vi "reserveResources.vi"(8 "error in (no error)":errorcluster, 10 "HWList":string[](array[string]), 11 "HWController in":refnum<class "HWController.lvclass">) -> (0 "error out":errorcluster, 3 "HWController out":refnum<class "HWController.lvclass">)   [LabVIEW 2011, in "Hardware.lvlib" / "HWControllers.lvlib" / "HWController.lvclass"]
uses:
  HWController.lvclass
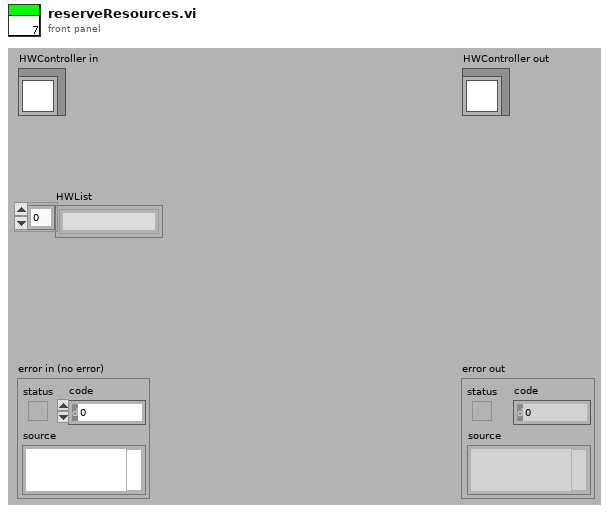
[diagram p1: front panel]
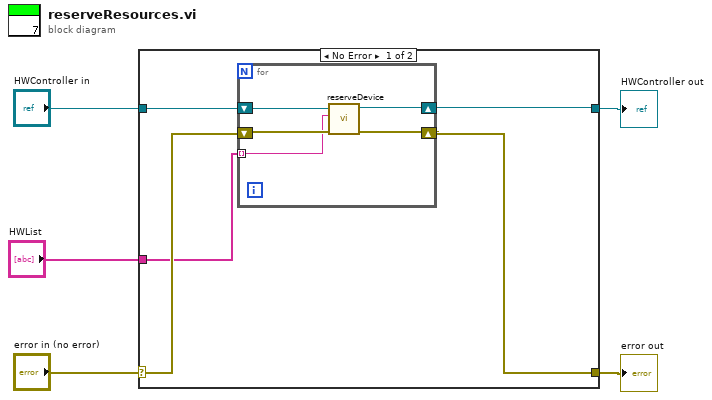
[diagram p0: block diagram]
diagram:
  n1 = case shown="No Error" "error in (no error)" {
    selector: "error in (no error)" -> [w8 w17]
    tunnel: [w7 w17] -> w4
    tunnel: [w9 w16] -> w2
    tunnel: "HWController in" -> [w10 w16]
    tunnel: "HWList" -> [w6 _]
    frame No Error {
      n2 = for {
        shift-right: [w14] -> w9
        shift-left: w10 -> [w15]
        shift-right: [w12] -> w7
        shift-left: w8 -> [w13]
        tunnel: w6 -> [w11] mode=indexing
        n3 = call "reserveDevice.vi"("error in (no error)"=w13, "deviceName"=w11, "HWController in"=w15) -> ("error out"=w12:errorcluster, "HWController out"=w14:refnum<class "HWController.lvclass">)  [unwired: 7 in]
      }
    }
    frame Error {
    }
  }
  "error out" <- w4
  "HWController out" <- w2
